vi "UDP Get Last Update Channel.vi"(8 "error in (no error)":errorcluster, 11 "E2E editor node in":refnum<data-value>) -> (0 "error out":errorcluster, 2 "channel out":refnum<class "TBM channel.lvclass">, 3 "E2E editor node out":refnum<data-value>)   [LabVIEW 2015, in "E2E Tag Exchange editor node.lvclass"]
uses:
  E2E Tag Exchange editor node.lvclass
  <vilib>/NI/Tag Bus Module Framework/channel/TBM channel.lvclass
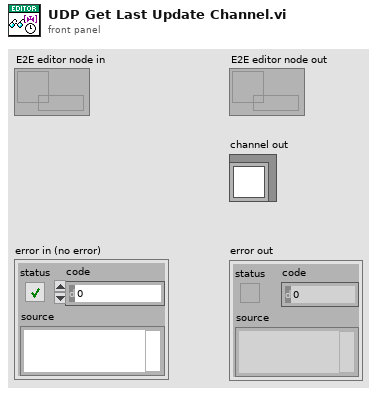
[diagram p1: front panel]
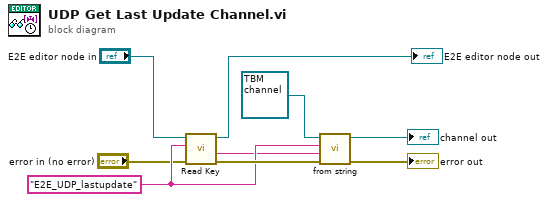
[diagram p0: block diagram]
diagram:
  w7 = "E2E_UDP_lastupdate" ("Key")
  n1 = call "Read Key.vi"("error in (no error)"="error in (no error)", "Key"=w7, "E2E editor node in"="E2E editor node in") -> ("error out"=w9:errorcluster, "Value"=w6:string, "E2E editor node out"=→"E2E editor node out":refnum<data-value>)  [unwired: 6 in]
  n2 = call-dynamic "from string.vi"("error in"=w9, "channel data"=w6, "identifier"=w7, "channel in"=refnum<class "TBM channel.lvclass"> refnum) -> ("error out"=→"error out":errorcluster, "channel out"=→"channel out":refnum<class "TBM channel.lvclass">)  [unwired: 6 in]
